vi "TB-Init Stimulus.vi"(0 "Exposure parameters":T3={"Low cutoff (kHz)"=0.0, "High cutoff (kHz)"=0.0, "Duration (min)"=0.0, "dB SPL"=0.0, "Waveform"=enum."Noise", "WAVfile"=path "", "refWav"=path "", "use mic correction"=FALSE, "micCorrFile"=path "", "Pistonphone Level (dB SPL)"=0.0, "Sampling rate (Hz)"=0.0, "Buffer length (s)"=0.0, "Stream mic"=FALSE, "Fine adjust"={"Max"=0.0, "Min"=0.0}, "Mic gain"=0.0, "atten"=0.0, "Allow Slack"=FALSE, "max starts"=0, "Freq (kHz)"=8.0, "Tma (s)"=0.0, "Streamed"=[], "Drive"="", "Speaker"="", "Mic"="", "Analysis"={"Method"=enum."Default", "resol (Hz)"=0.0, "nfreq"=0, "signal"=""}, "exposeAtten"=0.0, "Digital"=""}, 7 "Sampling rate (Hz)":dbl, 9 "Npts":i32, 11 "error in (no error)":errorcluster, 13 "Exposure":bool) -> (4 "state":T1, 15 "error out":errorcluster)   [LabVIEW 2020]
uses:
  Typedefs/TB-Parameters.ctl
  Typedefs/TB-Analysis Parameters.ctl
  Typedefs/TB-Stimulus State.ctl
  epl-vi-lib/Signal Synthesis VIs/4th Generation/Classes/SignalManager/SignalManager.lvclass
  <vilib>/sound2/lvsound2.llb/Sound File Refnum.ctl
  epl-vi-lib/Signal Synthesis VIs/4th Generation/Classes/Level/LevelUnits.ctl
  epl-vi-lib/Signal Synthesis VIs/4th Generation/Classes/Filter/Shape.ctl
  epl-vi-lib/Signal Synthesis VIs/4th Generation/Classes/Filter/Units.ctl
  epl-vi-lib/Signal Synthesis VIs/4th Generation/Classes/Filter/Filter.lvclass/Filter.ctl
  epl-vi-lib/Signal Synthesis VIs/4th Generation/Classes/Level/Level.lvclass/Level.ctl
  epl-vi-lib/Signal Synthesis VIs/4th Generation/Classes/Channel/Channel.lvclass/Channel.ctl
  epl-vi-lib/Signal Synthesis VIs/4th Generation/Classes/Waveforms/Tone/Tone.lvclass/Tone.ctl
  4c580b1c-7265-4c7e-a765-74f1412c170e.vi
  e934bc7d-9541-40f0-a8df-ff11fa5a53c0.vi
  epl-vi-lib/Signal Synthesis VIs/4th Generation/Classes/Level/Write Units.vi
  epl-vi-lib/Signal Synthesis VIs/4th Generation/Classes/Level/Write Level.vi
  epl-vi-lib/Signal Synthesis VIs/4th Generation/Classes/Filter/Write Type.vi
  epl-vi-lib/Signal Synthesis VIs/4th Generation/Classes/Filter/Write Units.vi
  epl-vi-lib/Signal Synthesis VIs/4th Generation/Classes/Filter/Write BW (kHz).vi
  epl-vi-lib/Signal Synthesis VIs/4th Generation/Classes/Filter/Write CF (kHz).vi
  epl-vi-lib/Signal Synthesis VIs/4th Generation/Classes/Channel/Write Waveform.vi
  epl-vi-lib/Signal Synthesis VIs/4th Generation/Classes/Channel/Write Level.vi
  epl-vi-lib/Signal Synthesis VIs/4th Generation/Classes/Channel/Write Filter.vi
  epl-vi-lib/Signal Synthesis VIs/4th Generation/Classes/Channel/Write Destination.vi
  epl-vi-lib/Signal Synthesis VIs/4th Generation/Classes/Waveforms/Tone/Write Frequency (kHz).vi
  epl-vi-lib/Signal Synthesis VIs/4th Generation/Classes/Waveforms/Noise/Noise.lvclass
  D:/Development/epl-vi-lib/Signal Synthesis VIs/4th Generation/Classes/Waveforms/Waveform/Waveform.lvclass
  epl-vi-lib/Signal Synthesis VIs/4th Generation/Classes/Waveforms/Tone/Tone.lvclass
  <vilib>/sound2/lvsound2.llb/Sound File Info (path).vi
  <vilib>/sound2/lvsound2.llb/Sound File Read Open.vi
  epl-vi-lib/Signal Synthesis VIs/4th Generation/Classes/Channel/Channel.lvclass
  epl-vi-lib/Signal Synthesis VIs/4th Generation/Classes/Level/Level.lvclass
  epl-vi-lib/Signal Synthesis VIs/4th Generation/Classes/Filter/Filter.lvclass
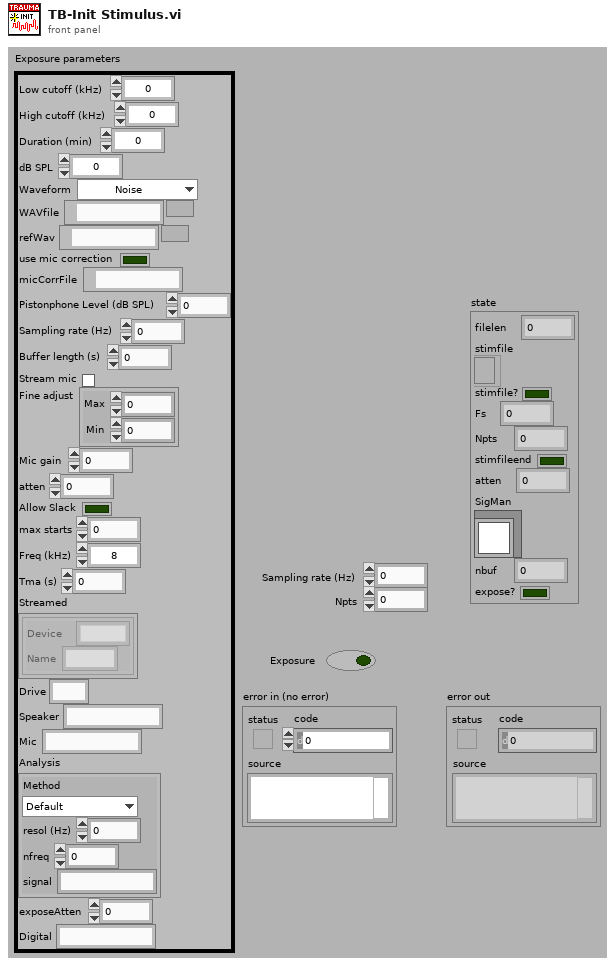
[diagram p1: front panel]
types:
  T1 = typedef "TB-Stimulus State.ctl" = cluster{"filelen":i32, "stimfile":T2, "stimfile?":bool, "Fs":dbl, "Npts":i32, "stimfileend":bool, "atten":dbl, "SigMan":refnum<class "SignalManager.lvclass">, "nbuf":i32, "expose?":bool}
  T2 = typedef "Sound File Refnum.ctl" = refnum<file>
  T3 = typedef "TB-Parameters.ctl" = cluster{"Low cutoff (kHz)":dbl, "High cutoff (kHz)":dbl, "Duration (min)":dbl, "dB SPL":dbl, "Waveform":enum16{"Noise", "File", "Tone"}, "WAVfile":path, "refWav":path, "use mic correction":bool, "micCorrFile":path, "Pistonphone Level (dB SPL)":dbl, "Sampling rate (Hz)":dbl, "Buffer length (s)":dbl, "Stream mic":bool, "Fine adjust":cluster{"Max":dbl, "Min":dbl}, "Mic gain":dbl, "atten":dbl, "Allow Slack":bool, "max starts":i32, "Freq (kHz)":dbl, "Tma (s)":dbl, "Streamed":cluster{"Device":string, "Name":string}[], "Drive":string, "Speaker":string, "Mic":string, "Analysis":T4, "exposeAtten":dbl, "Digital":string}
  T4 = typedef "TB-Analysis Parameters.ctl" = cluster{"Method":enum16{"Default", "Periodogram", "Cross-spectrum"}, "resol (Hz)":dbl, "nfreq":i32, "signal":string}
  T5 = typedef "Filter.lvclass/Units.ctl" = enum16{"Linear", "Octaves", "Min-Max"}
  T6 = typedef "Filter.lvclass/Shape.ctl" = enum16{"OFF", "Lowpass", "Highpass", "Bandpass", "Bandstop"}
  T7 = typedef "Level.lvclass/LevelUnits.ctl" = enum16{"dB atten", "dB SPL", "dB Vrms", "Volts", "dB mW", "mW", "dB HL", "dB SL"}
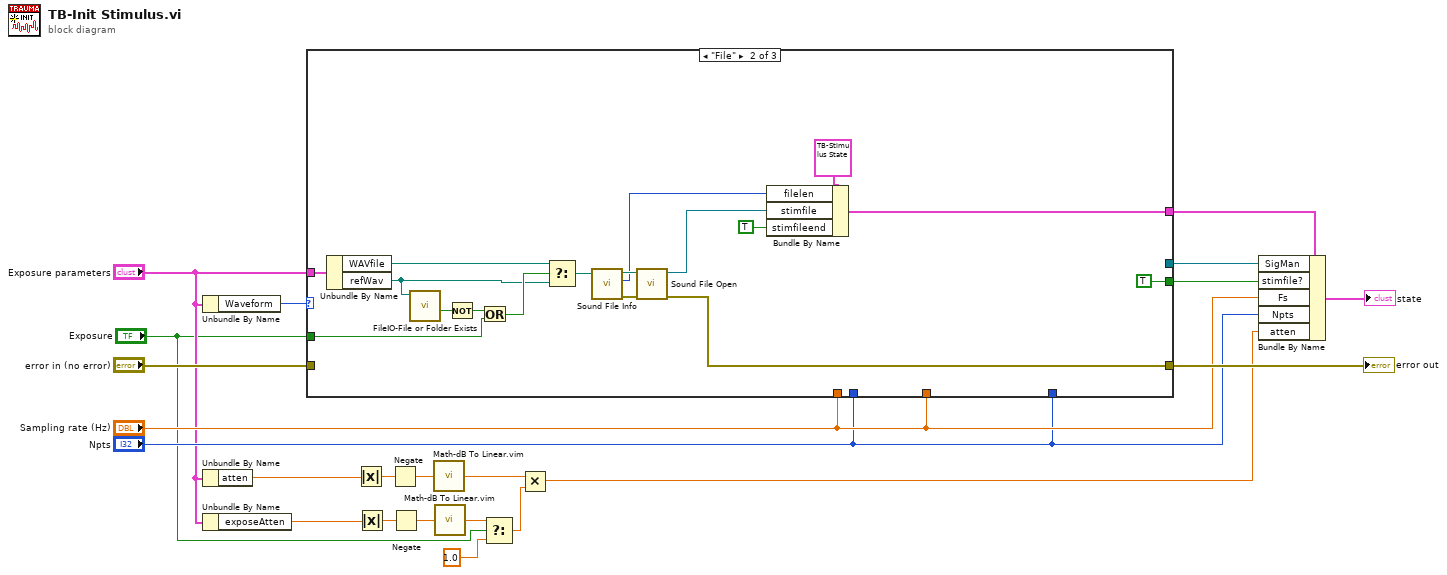
[diagram p0: block diagram]
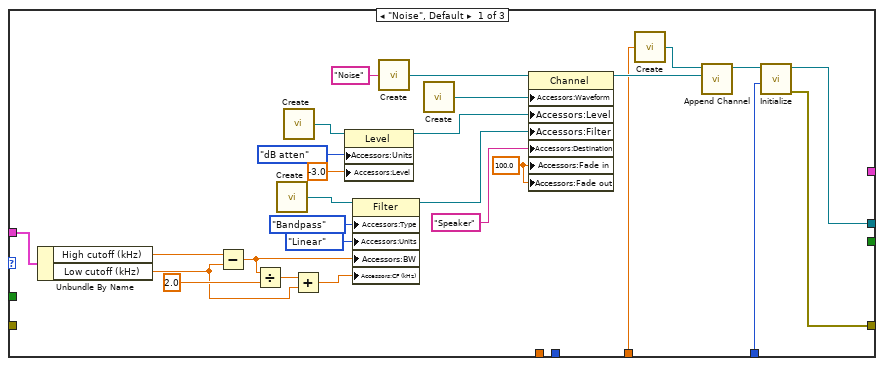
[diagram p2: hidden frame]
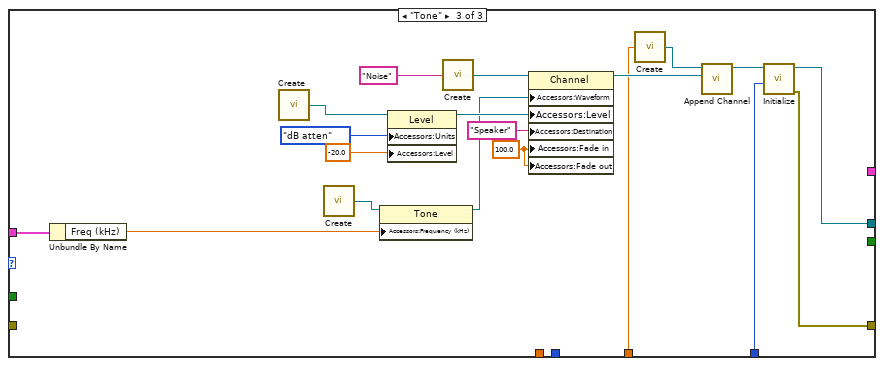
[diagram p3: hidden frame]
diagram:
  n1 = Unbundle By Name("Exposure parameters") -> ("Waveform"=w20:enum16{"Noise", "File", "Tone"})
  n2 = Unbundle By Name("Exposure parameters") -> ("atten"=w12:dbl)
  n3 = Unbundle By Name("Exposure parameters") -> ("exposeAtten"=w7:dbl)
  n4 = case shown="\"File\"" w20 {
    tunnel: "error in (no error)" -> [_ _ _]
    tunnel: [w26 w65 w70] -> w21
    tunnel: "Sampling rate (Hz)" -> [_ _ _]
    tunnel: "Exposure parameters" -> [w45 w66 w75]
    tunnel: [_ w61 _] -> w19
    tunnel: "Npts" -> [_ _ _]
    tunnel: [_ TRUE _] -> w18
    tunnel: "Exposure" -> [_ w57 _]
    tunnel: "Sampling rate (Hz)" -> [w28 _ w76]
    tunnel: "Npts" -> [w27 _ w71]
    tunnel: [w24 _ w68] -> w10
    frame "Noise", Default {
      w23 = 100.0 ("Fade in")
      n5 = Unbundle By Name(w45) -> ("High cutoff (kHz)"=w49:dbl, "Low cutoff (kHz)"=w46:dbl)
      n6 = Subtract(x=w49, y=w46) -> (x-y=w34:dbl)
      n7 = Divide(x=w34, y=2.0) -> (x/y=w47:dbl)
      n8 = call "Create.vi"() -> ("Filter"=w37:refnum<class "Filter.lvclass">)  [unwired: 15 in]
      n9 = call "Create.vi"() -> ("Level"=w41:refnum<class "Level.lvclass">)  [unwired: 15 in]
      n10 = Add(x=w47, y=w46) -> (x+y=w33:dbl)
      n11 = property class="Level"(reference=w41, "Accessors:Units"=LevelUnits."dB atten" ("Units"), "Accessors:Level"=-3.0 ("Level")) -> (reference out=w38:refnum<class "Level.lvclass">)  [unwired: 1 in, 1 out]
      n12 = property class="Filter"(reference=w37, "Accessors:Type"=Shape."Bandpass" ("Type"), "Accessors:Units"=Units."Linear" ("Units"), "Accessors:BW"=w34, "Accessors:CF (kHz)"=w33) -> (reference out=w32:refnum<class "Filter.lvclass">)  [unwired: 1 in, 1 out]
      n13 = call "Create.vi"("Name"="Noise") -> ("Channel"=w43:refnum<class "Channel.lvclass">)  [unwired: 14 in]
      n14 = call "Create.vi"() -> ("Noise"=w42:refnum<class "Noise.lvclass">)  [unwired: 15 in]
      n15 = property class="Channel"(reference=w43, "Accessors:Waveform"=w42, "Accessors:Level"=w38, "Accessors:Filter"=w32, "Accessors:Destination"="Speaker", "Accessors:Fade in"=w23, "Accessors:Fade out"=w23) -> (reference out=w30:refnum<class "Channel.lvclass">)  [unwired: 1 in, 1 out]
      n16 = call "Create.vi"("Fs (Hz)"=w28) -> ("SigMan"=w31:refnum<class "SignalManager.lvclass">)  [unwired: 14 in]
      n17 = call "Append Channel.vi"("Channel"=w30, "SignalManager in"=w31) -> ("SignalManager out"=w29:refnum<class "SignalManager.lvclass">)  [unwired: 8 in, 1 out]
      n18 = call "Initialize.vi"("Npts"=w27, "SigMan in"=w29) -> ("error out"=w26:errorcluster, "SigMan out"=w24:refnum<class "SignalManager.lvclass">)  [unwired: 8 in]
    }
    frame "File" {
      n19 = Unbundle By Name(w66) -> ("WAVfile"=w50:path, "refWav"=w55:path)
      n20 = call "FileIO-File or Folder Exists.vi"("path"=w55) -> ("Exists?"=w59:bool)  [unwired: 7 in, 3 out]
      n21 = Not(x=w59) -> (.not. x?=w58:bool)
      n22 = Or(x=w58, y=w57) -> (x .or. y?=w56:bool)
      n23 = Select(t=w50, s=w56, f=w55) -> (s? t:f=w54:path)
      n24 = call-poly <vilib>:"Sound File Info.vi"("path"=w54) -> ("error out"=w64:errorcluster, "total number of samples/ch"=w62:u32, "path out"=w63:path)  [unwired: 7 in, 1 out]
      n25 = call-poly <vilib>:"Sound File Open.vi"("error in (no error)"=w64, "path"=w63) -> ("error out"=w65:errorcluster, "sound file refnum"=w53:T2)  [unwired: 8 in]
      n26 = Bundle By Name(cluster=T1 {"filelen"=0, "stimfile"=refnum, "stimfile?"=FALSE, "Fs"=0.0, "Npts"=0, "stimfileend"=FALSE, "atten"=0.0, "SigMan"=refnum, "nbuf"=0, "expose?"=FALSE} ("state"), "filelen"=w62, "stimfile"=w53, "stimfileend"=TRUE) -> (w61:T1)
    }
    frame "Tone" {
      w67 = 100.0 ("Fade in")
      n27 = Unbundle By Name(w75) -> ("Freq (kHz)"=w73:dbl)
      n28 = call "Create.vi"() -> ("Level"=w83:refnum<class "Level.lvclass">)  [unwired: 15 in]
      n29 = call "Create.vi"() -> ("Tone"=w74:refnum<class "Tone.lvclass">)  [unwired: 15 in]
      n30 = property class="Tone"(reference=w74, "Accessors:Frequency (kHz)"=w73) -> (reference out=w72:refnum<class "Tone.lvclass">)  [unwired: 1 in, 1 out]
      n31 = property class="Level"(reference=w83, "Accessors:Units"=LevelUnits."dB atten" ("Units"), "Accessors:Level"=-20.0 ("Level")) -> (reference out=w80:refnum<class "Level.lvclass">)  [unwired: 1 in, 1 out]
      n32 = call "Create.vi"("Name"="Noise") -> ("Channel"=w84:refnum<class "Channel.lvclass">)  [unwired: 14 in]
      n33 = property class="Channel"(reference=w84, "Accessors:Waveform"=w72, "Accessors:Level"=w80, "Accessors:Destination"="Speaker", "Accessors:Fade in"=w67, "Accessors:Fade out"=w67) -> (reference out=w78:refnum<class "Channel.lvclass">)  [unwired: 1 in, 1 out]
      n34 = call "Create.vi"("Fs (Hz)"=w76) -> ("SigMan"=w79:refnum<class "SignalManager.lvclass">)  [unwired: 14 in]
      n35 = call "Append Channel.vi"("Channel"=w78, "SignalManager in"=w79) -> ("SignalManager out"=w77:refnum<class "SignalManager.lvclass">)  [unwired: 8 in, 1 out]
      n36 = call "Initialize.vi"("Npts"=w71, "SigMan in"=w77) -> ("error out"=w70:errorcluster, "SigMan out"=w68:refnum<class "SignalManager.lvclass">)  [unwired: 8 in]
    }
  }
  "error out" <- w21
  n37 = Absolute Value(x=w12) -> (abs(x)=w14:dbl)
  n38 = Absolute Value(x=w7) -> (abs(x)=w9:dbl)
  n39 = Negate(x=w14) -> (-x=w13:dbl)
  n40 = Negate(x=w9) -> (-x=w8:dbl)
  n41 = call "Math-dB To Linear.vim"("dB"=w13) -> ("linear"=w11:dbl)
  n42 = call "Math-dB To Linear.vim"("dB"=w8) -> ("linear"=w4:dbl)
  n43 = Select(t=w4, s="Exposure", f=1.0) -> (s? t:f=w3:dbl)
  n44 = Multiply(x=w11, y=w3) -> (x*y=w5:dbl)
  n45 = Bundle By Name(cluster=w19, "SigMan"=w10, "stimfile?"=w18, "Fs"="Sampling rate (Hz)", "Npts"="Npts", "atten"=w5) -> (→"state":T1)
